vi "TPNT_GetHelp.vi"(10 "name":string) -> (2 "help":string)   [LabVIEW 2016]
uses:
  TPNT_TP.ctl
  TPNT_Limits.ctl
  TPNT_Samples.ctl
  TPNT_Log.ctl
panel:
  in  "TPNT_TP":T1={"name"="", "type"="", "algor"=[], "update_rate"=0.0, "Limits"={"Alarm Type"="", "Lower "=0.0, "Upper"=0.0, "Nominal"=0.0, "outrange"=FALSE, "Check"=TRUE, "latch"=FALSE, "level"=""}, "Samples"={"samples"=0, "counter"=0, "Values"=[], "Current Value"="", "filter"="", "precision"=2}, "next_update"=0, "Status"="", "monitor"=TRUE, "error"=FALSE, "Log"={"log"=FALSE, "file"=path "", "type"="", "format"="", "updaterate"=0.0, "nex_update"=0, "mode"=""}, "permissions"="", "ID"=""} {"Log"."updaterate" format="%.2f"; "Samples"."Values" format="%.2f"; "Samples"."samples" min=1 step=1; "Limits"."Nominal" format="%.2f"; "Limits"."Upper" format="%.2f"; "Limits"."Lower" format="%.2f"; "update_rate" format="%.2f"}
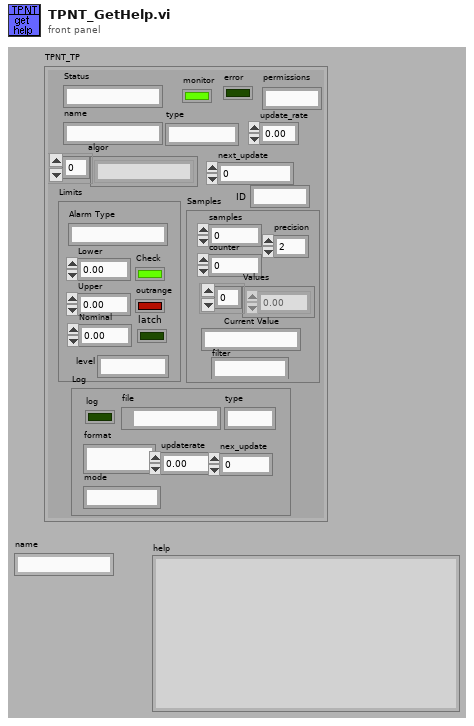
[diagram p1: front panel]
types:
  T1 = typedef "TPNT_TP.ctl" = cluster{"name":string, "type":string, "algor":string[], "update_rate":sgl, "Limits":T2, "Samples":T3, "next_update":u32, "Status":string, "monitor":bool, "error":bool, "Log":T4, "permissions":string, "ID":string}
  T2 = typedef "TPNT_Limits.ctl" = cluster{"Alarm Type":string, "Lower ":dbl, "Upper":dbl, "Nominal":dbl, "outrange":bool, "Check":bool, "latch":bool, "level":string}
  T3 = typedef "TPNT_Samples.ctl" = cluster{"samples":i32, "counter":i32, "Values":dbl[], "Current Value":string, "filter":string, "precision":u8}
  T4 = typedef "TPNT_Log.ctl" = cluster{"log":bool, "file":path, "type":string, "format":string, "updaterate":dbl, "nex_update":u32, "mode":string}
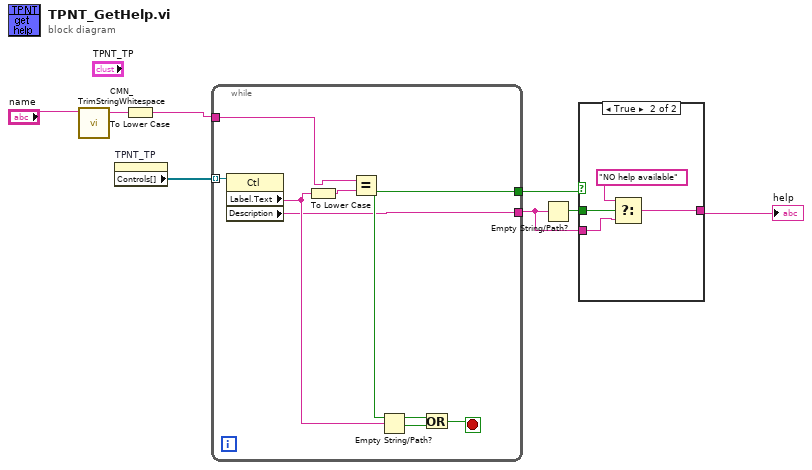
[diagram p0: block diagram]
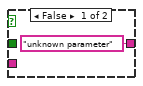
[diagram p2: hidden frame]
diagram:
  n1 = call "CMN_TrimStringWhitespace.vi"("string"="name") -> ("trimmed string"=w1:string)  [unwired: 1 in, 8 out]
  n2 = property on="TPNT_TP" class="Clust (strict)"() -> ("Controls[]"=w8:refnum<vi>[])  [unwired: 2 in, 2 out]
  n3 = To Lower Case(string=w1) -> (all lower case string=w7:string)
  n4 = while {
    tunnel: w8 -> [w16] mode=indexing
    tunnel: w7 -> [w13]
    tunnel: [w10] -> w6
    tunnel: [w9] -> w3
    stop <- w14 stop-if-true
    n5 = property class="Ctl"(reference=w16) -> ("Label.Text"=w12:string, "Description"=w9:string)  [unwired: 1 in, 2 out]
    n6 = To Lower Case(string=w12) -> (all lower case string=w11:string)
    n7 = Equal?(x=w13, y=w11) -> (x = y?=w10:bool)
    n8 = Empty String/Path?(string/path=w12) -> (empty?=w15:bool)
    n9 = Or(x=w10, y=w15) -> (x .or. y?=w14:bool)
  }
  n10 = Empty String/Path?(string/path=w3) -> (empty?=w4:bool)
  n11 = case shown="True" w6 {
    tunnel: ["unknown parameter" ("Desc") w19] -> w5
    tunnel: w4 -> [_ w21]
    tunnel: w3 -> [_ w20]
    frame False {
    }
    frame True {
      n12 = Select(t="NO help available", s=w21, f=w20) -> (s? t:f=w19:string)
    }
  }
  "help" <- w5
